vi "Dispatch Worker Mode Example(Sync).vi"() -> ()   [LabVIEW 2014]
uses:
  user.lib/_NEVSTOP/JKI State Machine ++/_Support/JKISMQ/_JKISMQFGV.vi
  user.lib/_NEVSTOP/JKI State Machine ++/JKI-State-Machine-Plus.lvlib
panel:
  in  "DoSth: DoA -@ Worker":bool
  in  "Name(\"\" to use uuid)":string="Event JKISM"
  out "State History":string
  in  "DoSth: DoA -> Worker":bool
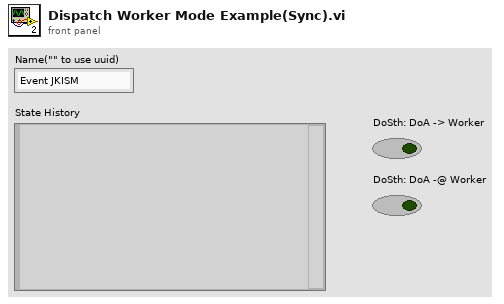
[diagram p1: front panel]
types:
  T1 = enum32{"Invalid", "Standard", "Closed", "Hidden", "Minimized", "Maximized"}
  T2 = enum32{"invalid app kind", "Development System", "Run Time System", "Student Edition", "Embedded LabVIEW", "Evaluation", "Custom"}
  T3 = cluster{"Core":cluster{"Current VI Reference":refnum<vi>, "Close Panel on Exit?":bool}, "Your Boolean data":bool, "Your string data":string}
  T4 = cluster{"Current VI Reference":refnum<vi>, "Close Panel on Exit?":bool}
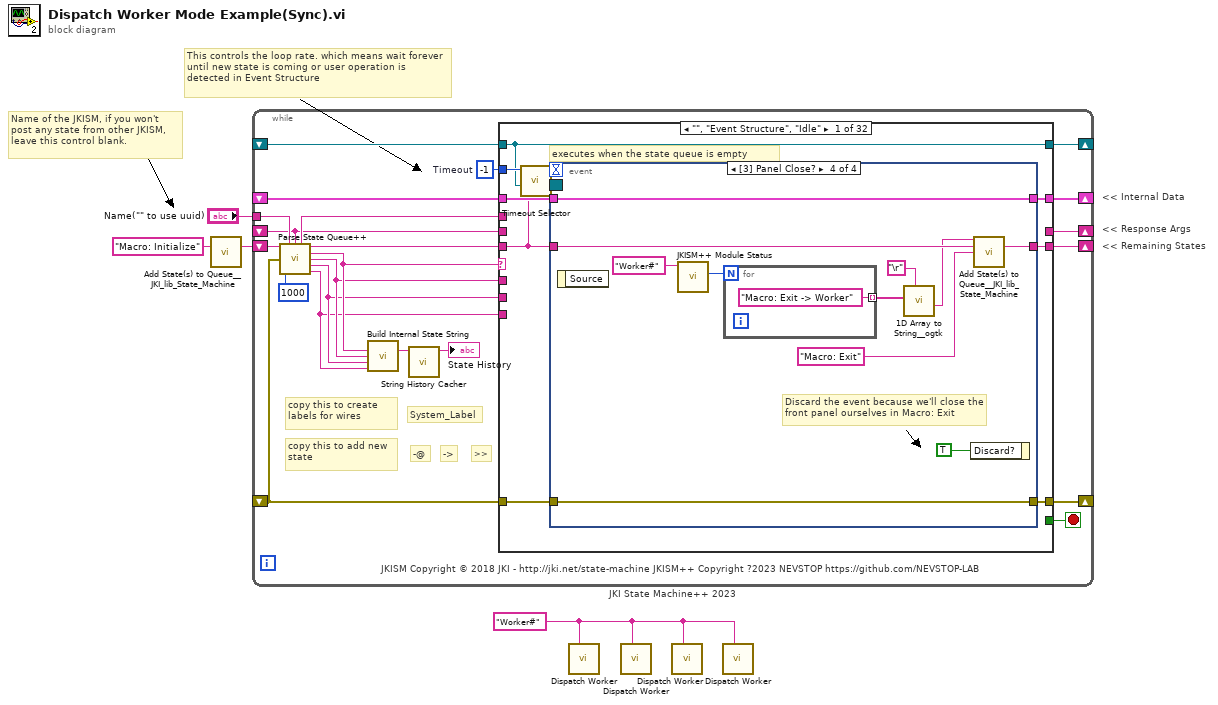
[diagram p0: block diagram]
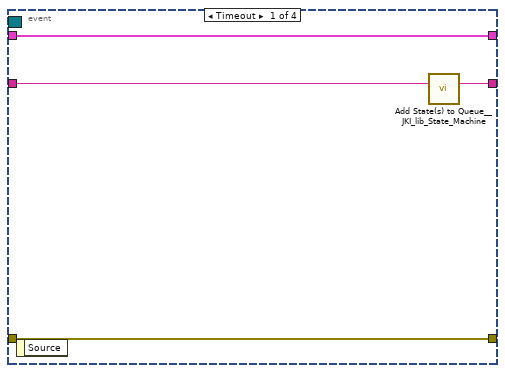
[diagram p2: hidden frame]
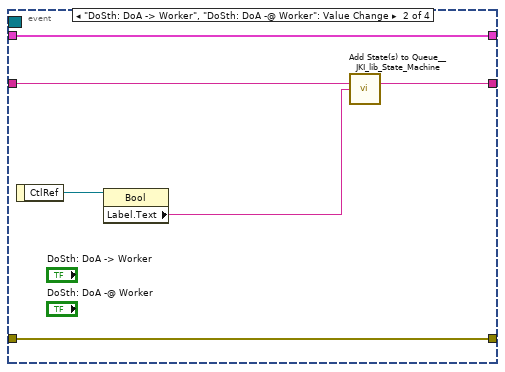
[diagram p3: hidden frame]
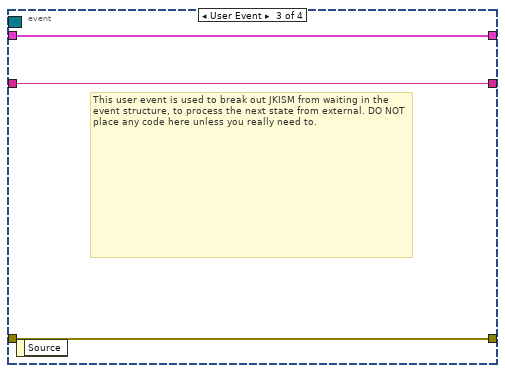
[diagram p4: hidden frame]
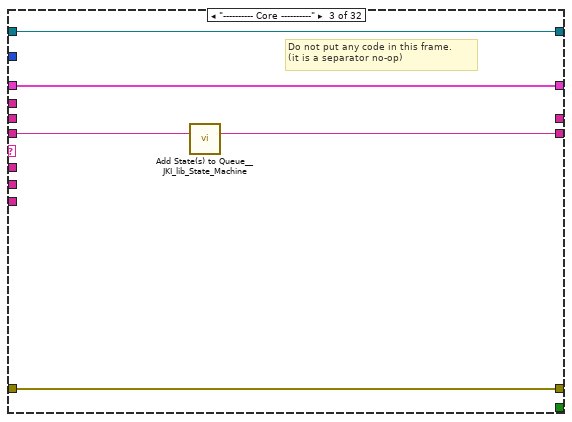
[diagram p6: hidden frame]
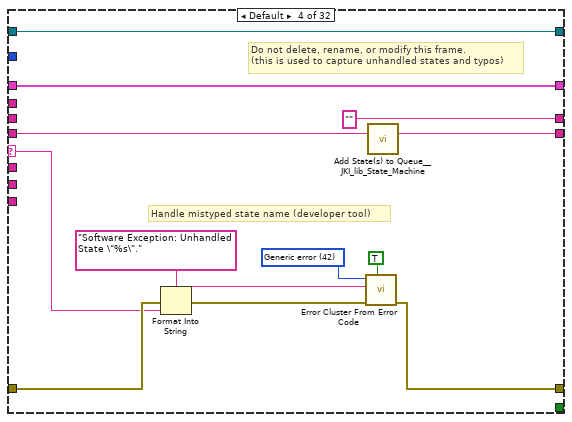
[diagram p7: hidden frame]
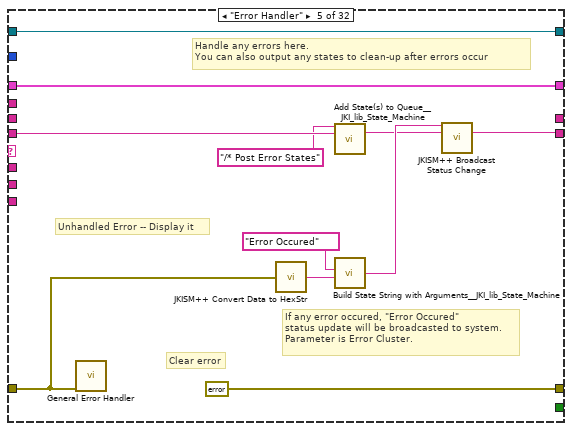
[diagram p8: hidden frame]
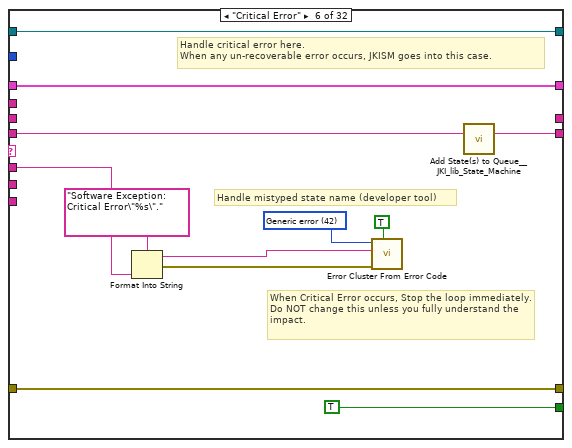
[diagram p9: hidden frame]
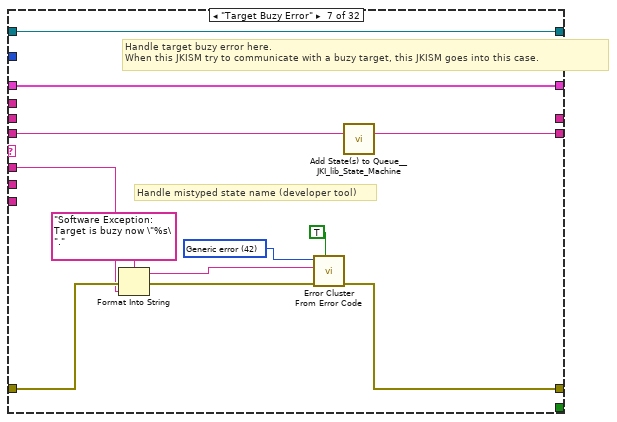
[diagram p10: hidden frame]
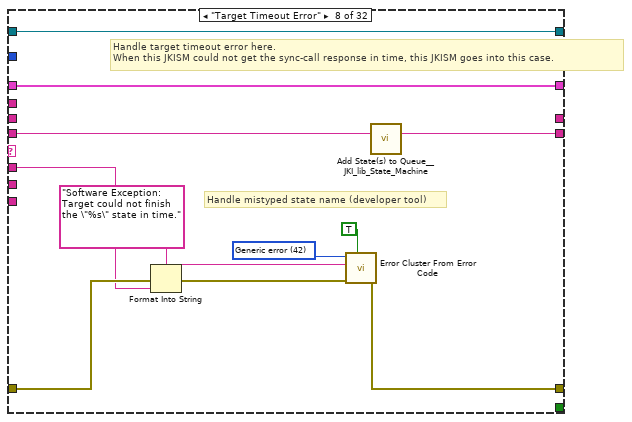
[diagram p11: hidden frame]
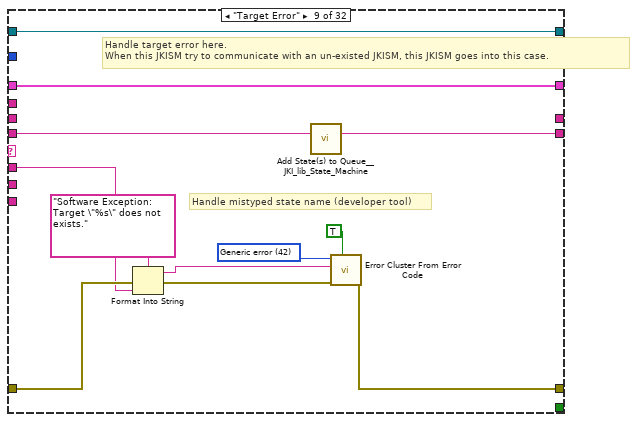
[diagram p12: hidden frame]
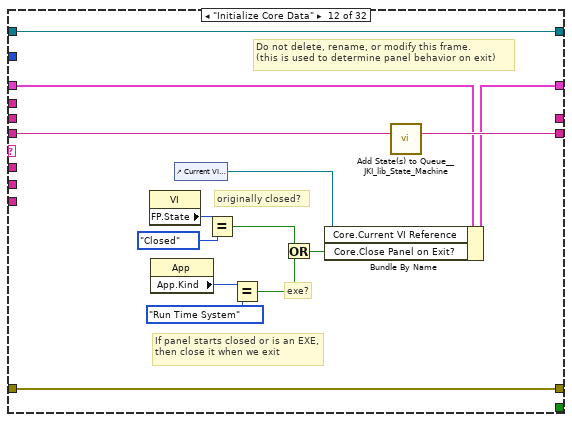
[diagram p15: hidden frame]
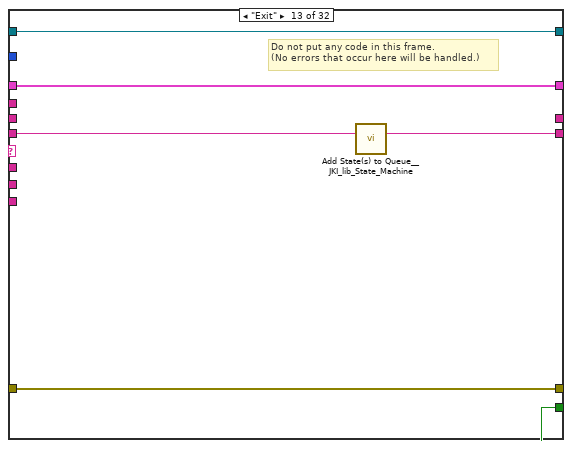
[diagram p16: hidden frame]
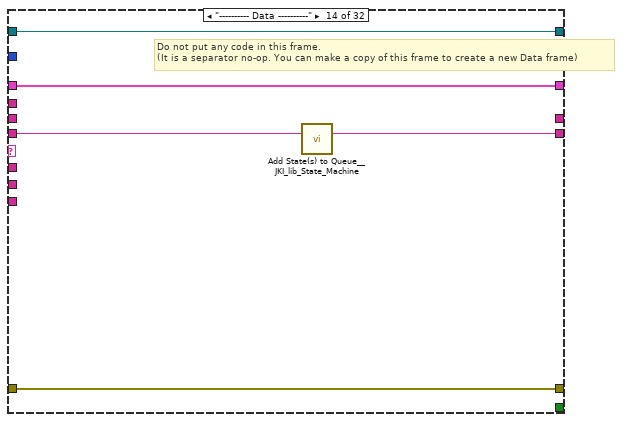
[diagram p17: hidden frame]
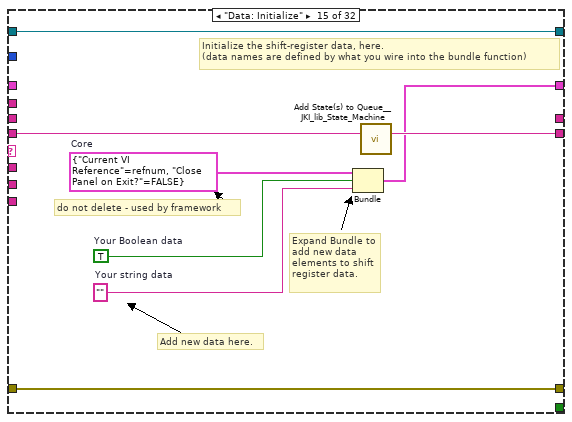
[diagram p18: hidden frame]
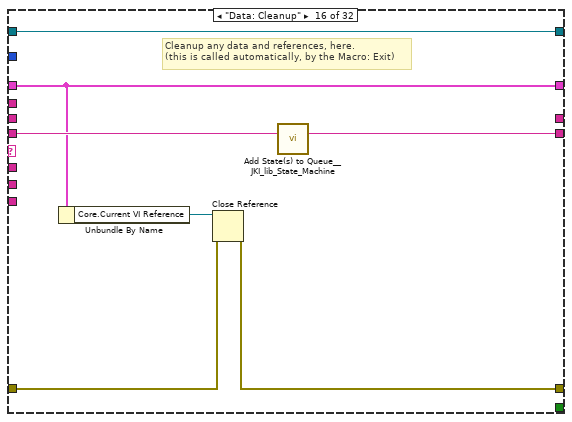
[diagram p19: hidden frame]
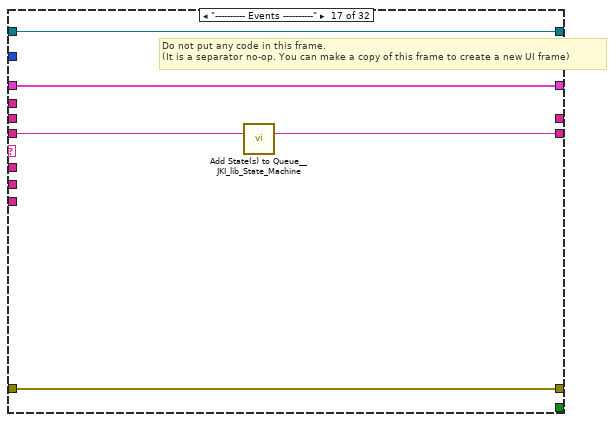
[diagram p20: hidden frame]
diagram:
  w1 = "Worker#" ("Name(\"\" to use uuid)")
  # "Name of the JKISM, if you won't post any state from other JKISM,  leave this control blank."
  # "This controls the loop rate. which means wait forever until new state is coming or user operation is detected in Event Structure"
  # "<< Internal Data"
  # "<< Response Args"
  # "<< Remaining States"
  n1 = call <vilib>:"Add State(s) to Queue__JKI_lib_State_Machine.vi"("State(s) in (\"\")"="Macro: Initialize") -> ("States Out"=w4:string)  [unwired: 14 in]
  n2 = while "JKI State Machine++ 2023" {
    shift-right: [w21] -> _
    shift-left: _ -> [w20]
    shift-right: [w24] -> _
    shift-left: _ -> [w18]
    shift-right: [w23] -> _
    shift-left: w4 -> [w25]
    tunnel: "Name(\"\" to use uuid)" -> [w13]
    shift-right: [w16] -> _
    shift-left: _ -> [w5]
    shift-right: [w15] -> _
    shift-left: _ -> [w14]
    stop <- w22 stop-if-true
    w19 = -1  # Timeout
    # "JKISM Copyright © 2018 JKI - http://jki.net/state-machine JKISM++ Copyright ?2023 NEVSTOP https://github.com/NEVSTOP-LAB"
    # "copy this to add new state"
    # ">>"
    # "->"
    # "-@"
    # "copy this to create labels for wires"
    # "System_Label"
    n3 = call "Parse State Queue++.vi"("State Queue"=w25, "Name(\"\" to use uuid)"=w13, "Response Arguments"=w5, "Error In (no error)"=w18, "Response Timeout(5000ms)"=1000 ("Response Timeout(1000ms)")) -> ("Name Used"=w6:string, "Remaining States"=w26:string, "Current State"=w10:string, "Arguments"=w9:string, "Argument - State"=w8:string, "From Who"=w7:string)  [unwired: 5 in]
    n4 = call "Build Internal State String.vi"("State"=w10, "Arguments (\"\")"=w9, "Arg-State (\"\")"=w8, "Source (\"\")"=w7) -> ("State with Arguments"=w11:string)  [unwired: 11 in]
    n5 = call "String History Cacher.vi"("String"=w11) -> ("String Cache"=→"State History":string)  [unwired: 10 in]
    n6 = case shown="\"\", \"Event Structure\", \"Idle\"" w10 {
      selector: w10 -> [_ _ _ w72 _ _ _ _ _ _ _ _ _ _ _ _ _ _ _ _ _ _ _ _ _ _ _ _ _ _ _ _]
      tunnel: w26 -> [w27 w63 w69 w76 w93 w103 w106 w123 w135 w144 w148 w163 w169 w174 w182 w189 w194 w200 w204 w210 w215 w222 w238 w308 w314 w325 w328 w333 w339 w347 w353 w359]
      tunnel: w9 -> [_ _ _ _ _ w96 w108 w119 w131 _ _ _ _ _ _ _ _ _ _ _ _ w217 w232 _ _ _ _ _ w336 _ _ _]
      tunnel: w20 -> [w34 w62 w66 w74 w91 w104 w110 w121 w133 w143 w147 w156 w167 w171 _ w184 w191 w199 w203 w207 w213 w220 w234 w305 w311 w322 w327 w332 w338 w344 w350 w356]
      tunnel: [w33 w64 w67 w78 errorcluster {"status"=FALSE, "code"=0, "source"=""} ("error out") w105 w113 w125 w137 w145 w149 w160 w166 w172 w179 w185 w192 w195 w202 w208 w212 w218 w235 w306 w312 w323 w329 w334 w340 w345 w351 w357] -> w24
      tunnel: w18 -> [w32 w64 w67 w77 w83 w105 w112 w124 w136 w145 w149 w160 w166 w172 w179 w186 w192 _ w205 w208 w212 w219 w236 w306 w312 w323 w329 w334 w340 w345 w351 w357]
      tunnel: [w35 w63 w68 w75 w84 w102 w111 w122 w134 w144 w148 w162 w168 w173 w181 w188 w193 w200 w204 w209 w214 w221 w237 w307 w313 w324 w328 w333 w339 w346 w352 w358] -> w23
      tunnel: [_ _ _ _ _ TRUE _ _ _ _ _ _ TRUE _ _ _ _ _ _ _ _ _ _ _ _ _ _ _ _ _ _ _] -> w22
      tunnel: [w31 w62 w66 w74 w91 w104 w110 w121 w133 w143 w147 w161 w167 w171 w180 w184 w191 w199 w203 w207 w213 w220 w234 w305 w311 w322 w327 w332 w338 w344 w350 w356] -> w21
      tunnel: w19 -> [w30 _ _ _ _ _ _ _ _ _ _ _ _ _ _ _ _ _ _ _ _ _ _ _ _ _ _ _ _ _ _ _]
      tunnel: w7 -> [_ _ _ _ _ _ _ _ _ _ _ _ _ _ _ _ _ _ _ _ _ _ _ _ _ _ _ _ _ _ _ _]
      tunnel: w8 -> [_ _ _ _ _ _ _ _ _ _ _ _ _ _ _ _ _ _ _ _ _ _ _ _ _ _ _ _ _ _ _ _]
      tunnel: [_ _ _ "" _ _ _ _ _ _ _ _ _ _ _ _ _ _ _ _ _ _ _ _ _ _ _ "API1 Response" w335 _ "DoA Finished" "DoB Finished"] -> w16
      tunnel: [w29 w61 w65 w70 w89 w94 w107 w118 w130 w142 w146 w150 w164 w170 w175 w183 w190 w198 w201 w206 w211 w216 w231 w304 w309 w315 w326 w331 w337 w343 w349 w355] -> w15
      tunnel: w14 -> [w29 w61 w65 w70 w89 w94 w107 w118 w130 w142 w146 w150 w164 w170 w175 w183 w190 _ w201 w206 w211 w216 w231 w304 w309 w315 w326 w331 w337 w343 w349 w355]
      tunnel: w6 -> [_ _ _ _ _ _ _ _ _ _ _ _ _ _ _ _ _ w197 _ _ _ _ _ _ _ _ _ _ _ _ _ _]
      tunnel: w5 -> [_ _ _ _ _ _ _ _ _ _ _ _ _ _ _ _ _ _ _ _ _ _ _ _ _ _ _ _ _ _ _ _]
      frame "", "Event Structure", "Idle" {
        # "executes when the state queue is empty"
        n7 = call "Timeout Selector.vi"("Remaining States"=w27, "Timeout Expected"=w30) -> ("Timeout"=w28:i32)  [unwired: 5 in]
        n8 = event shown="[3] Panel Close?" {
          selector: w29 -> [_ _ _ _]
          dyn-events: _ -> [_ _ _ _]
          timeout: w28 -> [_ _ _ _]
          tunnel: w27 -> [w39 w43 w47 w59]
          tunnel: [w38 w42 w47 w58] -> w35
          tunnel: w34 -> [w36 w44 w48 w56]
          tunnel: [w37 w45 w46 w57] -> w33
          tunnel: w32 -> [w37 w45 w46 w57]
          tunnel: [w36 w44 w48 w56] -> w31
          event Timeout {
            n9 = event-data() -> ()  [unwired: 1 in, 1 out]
            n10 = call <vilib>:"Add State(s) to Queue__JKI_lib_State_Machine.vi"("State(s) in (\"\")"=w39) -> ("States Out"=w38:string)  [unwired: 14 in]
          }
          event "DoSth: DoA -> Worker", "DoSth: DoA -@ Worker": Value Change {
            n11 = event-data() -> ("CtlRef"=w41:refnum<vi>)  [unwired: 1 in]
            n12 = property class="Bool"(reference=w41) -> ("Label.Text"=w40:string)  [unwired: 1 in, 2 out]
            n13 = call <vilib>:"Add State(s) to Queue__JKI_lib_State_Machine.vi"("State(s) in (\"\")"=w43, "State(s) at Back (\"\")"=w40) -> ("States Out"=w42:string)  [unwired: 13 in]
          }
          event User Event {
            # "This user event is used to break out JKISM from waiting in the event structure, to process the next state from external. DO NOT place any code here unless you really need to."
            n14 = event-data() -> ()  [unwired: 1 in, 1 out]
          }
          event Panel Close? {
            # "Discard the event because we'll close the front panel ourselves in Macro: Exit"
            n15 = event-data() -> ()  [unwired: 1 in, 1 out]
            n16 = call "JKISM++ Module Status.vi"("Name(\"\" to use uuid) in"="Worker#" ("Name(\"\" to use uuid)")) -> ("#AsWorker"=w53:i32)  [unwired: 7 in, 3 out]
            n17 = for {
              N: w53 -> [_]
              tunnel: ["Macro: Exit -> Worker"] -> w52 mode=indexing
            }
            n18 = call <userlib>:"1D Array to String__ogtk.vi"("delimiter (Tab)"="\r", "Array of Strings"=w52) -> ("delimited string"=w51:string)  [unwired: 9 in]
            n19 = event-data("Discard?"=TRUE) -> ()  [unwired: 1 in, 1 out]
            n20 = call <vilib>:"Add State(s) to Queue__JKI_lib_State_Machine.vi"("State(s) in Front (\"\")"=w51, "State(s) in (\"\")"=w59, "State(s) at Back (\"\")"="Macro: Exit") -> ("States Out"=w58:string)  [unwired: 12 in]
          }
        }
      }
      frame "JKISM++ Documentation" {
        # "JKISM++ Documentation"
        # "State Syntax:\nStateCategory: State >> Argument -@ JKISMName\nStateCategory: State >> Argument -> JKISMName\n\nLine Terminator: Line feed"
        # "Commenting:\nTo add a comment use \"//\" or \"#\" and all text to the right will be ignored\nCommenting Example:\nUI: Initialize // This initializes the UI\n# This whole line is a comment\n// Another comment line"
      }
      frame "---------- Core ----------" {
        # "Do not put any code in this frame.\n(it is a separator no-op)"
        n21 = call <vilib>:"Add State(s) to Queue__JKI_lib_State_Machine.vi"("State(s) in (\"\")"=w69) -> ("States Out"=w68:string)  [unwired: 14 in]
      }
      frame Default {
        w81 = 42 items=["No error", "Argument error", "Memory is full", "Out of zone", "End of file", "File already open", "Generic file I/O error", "File not found", "File permission error", "Disk is full", "Duplicate path", "Too many files open", "System feature not enabled", "Resource file not found", "Cannot add resource", "Resource not found", "Image not found", "Image memory error", "Pen does not exist", "Config type invalid", "Config token not found", "Config parse error", "Config memory error", "Bad external code format", "Bad external code offset", "External code not present", "Null window", "Destroy window error", "Null menu", "Print aborted", "Bad print record", "Print driver error", "Windows error during printing", "Memory error during printing", "Print dialog error", "Generic print error", "Invalid device refnum", "Device not found", "Device parameter error", "Device unit error", "Cannot open device", "Device call aborted", "Generic error", "Cancelled by user", "Object ID too low", "Object ID too high", "Object not in heap", "Unknown heap", "Unknown object (invalid DefProc)", "Unknown object (DefProc not in table)", "Message out of range", "Invalid (null) method", "Unknown message", "Manager call not supported", "Bad address", "Network operation in progress", "Network operation timed out", "Connection is busy", "Network attribute not supported", "Network error", "Address in use", "System out of memory", "Connection aborted", "Connection refused", "Not connected", "Already connected", "Connection closed", "Initialization error (interapplication manager)", "Bad occurrence", "Wait on unbound occurrence handler", "Occurrence queue overflow", "Datalog type conflict", "Unused", "Unrecognized type (interapplication manager)", "Memory corrupt", "Failed to make temporary DLL", "Old CIN version", "Drag socket not found", "Failed to load drop-object", "Failed to register OLE object", "Failed to release OLE object", "Format specifier type mismatch", "Unknown format specifier", "Too few format specifiers", "Too many format specifiers", "Scan failed", "Newer CIN version", "Error converting to variant", "Runtime menu error", "Password tampered", "Variant attribute not found", "Incompatible variant data type", "Event data is not available", "Event Store is not present", "Occurrence is not found", "Event Queue is not created", "Event info is not available", "Refnum passed is NULL", "Error retrieving Class GUID", "Error retrieving CoClass GUID", "Error retrieving TypeLib GUID.", "Bad built application magic bytes.", "Specific driver is different from the specific driver associated with the Logical Name.", "There is no session opened to the class driver.", "Max Error", "MAX - Error with config objects", "MAX - Error loading configuration", "MAX - Group not supported"]
        # "Do not delete, rename, or modify this frame.\n(this is used to capture unhandled states and typos)"
        # "Handle mistyped state name (developer tool)"
        n22 = Format Into String(format string="Software Exception: Unhandled State \"%s\"." ("message"), error in=w77, w72) -> (resulting string=w80:string, error out=w79:errorcluster)  [unwired: 1 in]
        n23 = call <vilib>:"Error Cluster From Error Code.vi"("show call chain? (False)"=TRUE, "error in (no error)"=w79, "error message (\"\")"=w80, "error code (0)"=w81) -> ("error out"=w78:errorcluster)  [unwired: 5 in]
        n24 = call <vilib>:"Add State(s) to Queue__JKI_lib_State_Machine.vi"("State(s) in (\"\")"=w76) -> ("States Out"=w75:string)  [unwired: 14 in]
      }
      frame "Error Handler" {
        # "If any error occured, \"Error Occured\" \nstatus update will be broadcasted to system.\nParameter is Error Cluster."
        # "Unhandled Error -- Display it"
        # "Handle any errors here.\nYou can also output any states to clean-up after errors occur"
        # "Clear error"
        n25 = call <vilib>:"General Error Handler.vi"("error in (no error)"=w83) -> ()  [unwired: 10 in, 5 out]
        n26 = call "JKISM++ Convert Data to HexStr.vi"("Variant"=w83) -> ("HEX String (0-9,A-F)"=w87:string)  [unwired: 8 in]
        n27 = call <vilib>:"Add State(s) to Queue__JKI_lib_State_Machine.vi"("State(s) in Front (\"\")"="/* Post Error States", "State(s) in (\"\")"=w93) -> ("States Out"=w85:string)  [unwired: 13 in]
        n28 = call <vilib>:"Build State String with Arguments__JKI_lib_State_Machine.vi"("Arguments (\"\")"=w87, "State"="Error Occured" ("Status with Arguments")) -> ("State with Arguments"=w86:string)  [unwired: 4 in]
        n29 = call "JKISM++ Broadcast Status Change.vi"("Status with Arguments"=w86, "State(s) in (\"\")"=w85) -> ("States Out"=w84:string)  [unwired: 13 in]
      }
      frame "Critical Error" {
        w100 = 42 items=["No error", "Argument error", "Memory is full", "Out of zone", "End of file", "File already open", "Generic file I/O error", "File not found", "File permission error", "Disk is full", "Duplicate path", "Too many files open", "System feature not enabled", "Resource file not found", "Cannot add resource", "Resource not found", "Image not found", "Image memory error", "Pen does not exist", "Config type invalid", "Config token not found", "Config parse error", "Config memory error", "Bad external code format", "Bad external code offset", "External code not present", "Null window", "Destroy window error", "Null menu", "Print aborted", "Bad print record", "Print driver error", "Windows error during printing", "Memory error during printing", "Print dialog error", "Generic print error", "Invalid device refnum", "Device not found", "Device parameter error", "Device unit error", "Cannot open device", "Device call aborted", "Generic error", "Cancelled by user", "Object ID too low", "Object ID too high", "Object not in heap", "Unknown heap", "Unknown object (invalid DefProc)", "Unknown object (DefProc not in table)", "Message out of range", "Invalid (null) method", "Unknown message", "Manager call not supported", "Bad address", "Network operation in progress", "Network operation timed out", "Connection is busy", "Network attribute not supported", "Network error", "Address in use", "System out of memory", "Connection aborted", "Connection refused", "Not connected", "Already connected", "Connection closed", "Initialization error (interapplication manager)", "Bad occurrence", "Wait on unbound occurrence handler", "Occurrence queue overflow", "Datalog type conflict", "Unused", "Unrecognized type (interapplication manager)", "Memory corrupt", "Failed to make temporary DLL", "Old CIN version", "Drag socket not found", "Failed to load drop-object", "Failed to register OLE object", "Failed to release OLE object", "Format specifier type mismatch", "Unknown format specifier", "Too few format specifiers", "Too many format specifiers", "Scan failed", "Newer CIN version", "Error converting to variant", "Runtime menu error", "Password tampered", "Variant attribute not found", "Incompatible variant data type", "Event data is not available", "Event Store is not present", "Occurrence is not found", "Event Queue is not created", "Event info is not available", "Refnum passed is NULL", "Error retrieving Class GUID", "Error retrieving CoClass GUID", "Error retrieving TypeLib GUID.", "Bad built application magic bytes.", "Specific driver is different from the specific driver associated with the Logical Name.", "There is no session opened to the class driver.", "Max Error", "MAX - Error with config objects", "MAX - Error loading configuration", "MAX - Group not supported"]
        # "Handle critical error here.\nWhen any un-recoverable error occurs, JKISM goes into this case."
        # "When Critical Error occurs, Stop the loop immediately. Do NOT change this unless you fully understand the impact."
        # "Handle mistyped state name (developer tool)"
        n30 = Format Into String(format string="Software Exception: Critical Error\"%s\"." ("message"), w96) -> (resulting string=w99:string, error out=w98:errorcluster)  [unwired: 2 in]
        n31 = call <vilib>:"Error Cluster From Error Code.vi"("show call chain? (False)"=TRUE, "error in (no error)"=w98, "error message (\"\")"=w99, "error code (0)"=w100) -> ()  [unwired: 5 in, 1 out]
        n32 = call <vilib>:"Add State(s) to Queue__JKI_lib_State_Machine.vi"("State(s) in (\"\")"=w103) -> ("States Out"=w102:string)  [unwired: 14 in]
      }
      frame "Target Buzy Error" {
        w116 = 42 items=["No error", "Argument error", "Memory is full", "Out of zone", "End of file", "File already open", "Generic file I/O error", "File not found", "File permission error", "Disk is full", "Duplicate path", "Too many files open", "System feature not enabled", "Resource file not found", "Cannot add resource", "Resource not found", "Image not found", "Image memory error", "Pen does not exist", "Config type invalid", "Config token not found", "Config parse error", "Config memory error", "Bad external code format", "Bad external code offset", "External code not present", "Null window", "Destroy window error", "Null menu", "Print aborted", "Bad print record", "Print driver error", "Windows error during printing", "Memory error during printing", "Print dialog error", "Generic print error", "Invalid device refnum", "Device not found", "Device parameter error", "Device unit error", "Cannot open device", "Device call aborted", "Generic error", "Cancelled by user", "Object ID too low", "Object ID too high", "Object not in heap", "Unknown heap", "Unknown object (invalid DefProc)", "Unknown object (DefProc not in table)", "Message out of range", "Invalid (null) method", "Unknown message", "Manager call not supported", "Bad address", "Network operation in progress", "Network operation timed out", "Connection is busy", "Network attribute not supported", "Network error", "Address in use", "System out of memory", "Connection aborted", "Connection refused", "Not connected", "Already connected", "Connection closed", "Initialization error (interapplication manager)", "Bad occurrence", "Wait on unbound occurrence handler", "Occurrence queue overflow", "Datalog type conflict", "Unused", "Unrecognized type (interapplication manager)", "Memory corrupt", "Failed to make temporary DLL", "Old CIN version", "Drag socket not found", "Failed to load drop-object", "Failed to register OLE object", "Failed to release OLE object", "Format specifier type mismatch", "Unknown format specifier", "Too few format specifiers", "Too many format specifiers", "Scan failed", "Newer CIN version", "Error converting to variant", "Runtime menu error", "Password tampered", "Variant attribute not found", "Incompatible variant data type", "Event data is not available", "Event Store is not present", "Occurrence is not found", "Event Queue is not created", "Event info is not available", "Refnum passed is NULL", "Error retrieving Class GUID", "Error retrieving CoClass GUID", "Error retrieving TypeLib GUID.", "Bad built application magic bytes.", "Specific driver is different from the specific driver associated with the Logical Name.", "There is no session opened to the class driver.", "Max Error", "MAX - Error with config objects", "MAX - Error loading configuration", "MAX - Group not supported"]
        # "Handle target buzy error here.\nWhen this JKISM try to communicate with a buzy target, this JKISM goes into this case."
        # "Handle mistyped state name (developer tool)"
        n33 = Format Into String(format string="Software Exception: Target is buzy now \"%s\"." ("message"), error in=w112, w108) -> (resulting string=w115:string, error out=w114:errorcluster)  [unwired: 1 in]
        n34 = call <vilib>:"Error Cluster From Error Code.vi"("show call chain? (False)"=TRUE, "error in (no error)"=w114, "error message (\"\")"=w115, "error code (0)"=w116) -> ("error out"=w113:errorcluster)  [unwired: 5 in]
        n35 = call <vilib>:"Add State(s) to Queue__JKI_lib_State_Machine.vi"("State(s) in (\"\")"=w106) -> ("States Out"=w111:string)  [unwired: 14 in]
      }
      frame "Target Timeout Error" {
        w128 = 42 items=["No error", "Argument error", "Memory is full", "Out of zone", "End of file", "File already open", "Generic file I/O error", "File not found", "File permission error", "Disk is full", "Duplicate path", "Too many files open", "System feature not enabled", "Resource file not found", "Cannot add resource", "Resource not found", "Image not found", "Image memory error", "Pen does not exist", "Config type invalid", "Config token not found", "Config parse error", "Config memory error", "Bad external code format", "Bad external code offset", "External code not present", "Null window", "Destroy window error", "Null menu", "Print aborted", "Bad print record", "Print driver error", "Windows error during printing", "Memory error during printing", "Print dialog error", "Generic print error", "Invalid device refnum", "Device not found", "Device parameter error", "Device unit error", "Cannot open device", "Device call aborted", "Generic error", "Cancelled by user", "Object ID too low", "Object ID too high", "Object not in heap", "Unknown heap", "Unknown object (invalid DefProc)", "Unknown object (DefProc not in table)", "Message out of range", "Invalid (null) method", "Unknown message", "Manager call not supported", "Bad address", "Network operation in progress", "Network operation timed out", "Connection is busy", "Network attribute not supported", "Network error", "Address in use", "System out of memory", "Connection aborted", "Connection refused", "Not connected", "Already connected", "Connection closed", "Initialization error (interapplication manager)", "Bad occurrence", "Wait on unbound occurrence handler", "Occurrence queue overflow", "Datalog type conflict", "Unused", "Unrecognized type (interapplication manager)", "Memory corrupt", "Failed to make temporary DLL", "Old CIN version", "Drag socket not found", "Failed to load drop-object", "Failed to register OLE object", "Failed to release OLE object", "Format specifier type mismatch", "Unknown format specifier", "Too few format specifiers", "Too many format specifiers", "Scan failed", "Newer CIN version", "Error converting to variant", "Runtime menu error", "Password tampered", "Variant attribute not found", "Incompatible variant data type", "Event data is not available", "Event Store is not present", "Occurrence is not found", "Event Queue is not created", "Event info is not available", "Refnum passed is NULL", "Error retrieving Class GUID", "Error retrieving CoClass GUID", "Error retrieving TypeLib GUID.", "Bad built application magic bytes.", "Specific driver is different from the specific driver associated with the Logical Name.", "There is no session opened to the class driver.", "Max Error", "MAX - Error with config objects", "MAX - Error loading configuration", "MAX - Group not supported"]
        # "Handle target timeout error here.\nWhen this JKISM could not get the sync-call response in time, this JKISM goes into this case."
        # "Handle mistyped state name (developer tool)"
        n36 = Format Into String(format string="Software Exception: Target could not finish the \"%s\" state in time." ("message"), error in=w124, w119) -> (resulting string=w127:string, error out=w126:errorcluster)  [unwired: 1 in]
        n37 = call <vilib>:"Error Cluster From Error Code.vi"("show call chain? (False)"=TRUE, "error in (no error)"=w126, "error message (\"\")"=w127, "error code (0)"=w128) -> ("error out"=w125:errorcluster)  [unwired: 5 in]
        n38 = call <vilib>:"Add State(s) to Queue__JKI_lib_State_Machine.vi"("State(s) in (\"\")"=w123) -> ("States Out"=w122:string)  [unwired: 14 in]
      }
      frame "Target Error" {
        w140 = 42 items=["No error", "Argument error", "Memory is full", "Out of zone", "End of file", "File already open", "Generic file I/O error", "File not found", "File permission error", "Disk is full", "Duplicate path", "Too many files open", "System feature not enabled", "Resource file not found", "Cannot add resource", "Resource not found", "Image not found", "Image memory error", "Pen does not exist", "Config type invalid", "Config token not found", "Config parse error", "Config memory error", "Bad external code format", "Bad external code offset", "External code not present", "Null window", "Destroy window error", "Null menu", "Print aborted", "Bad print record", "Print driver error", "Windows error during printing", "Memory error during printing", "Print dialog error", "Generic print error", "Invalid device refnum", "Device not found", "Device parameter error", "Device unit error", "Cannot open device", "Device call aborted", "Generic error", "Cancelled by user", "Object ID too low", "Object ID too high", "Object not in heap", "Unknown heap", "Unknown object (invalid DefProc)", "Unknown object (DefProc not in table)", "Message out of range", "Invalid (null) method", "Unknown message", "Manager call not supported", "Bad address", "Network operation in progress", "Network operation timed out", "Connection is busy", "Network attribute not supported", "Network error", "Address in use", "System out of memory", "Connection aborted", "Connection refused", "Not connected", "Already connected", "Connection closed", "Initialization error (interapplication manager)", "Bad occurrence", "Wait on unbound occurrence handler", "Occurrence queue overflow", "Datalog type conflict", "Unused", "Unrecognized type (interapplication manager)", "Memory corrupt", "Failed to make temporary DLL", "Old CIN version", "Drag socket not found", "Failed to load drop-object", "Failed to register OLE object", "Failed to release OLE object", "Format specifier type mismatch", "Unknown format specifier", "Too few format specifiers", "Too many format specifiers", "Scan failed", "Newer CIN version", "Error converting to variant", "Runtime menu error", "Password tampered", "Variant attribute not found", "Incompatible variant data type", "Event data is not available", "Event Store is not present", "Occurrence is not found", "Event Queue is not created", "Event info is not available", "Refnum passed is NULL", "Error retrieving Class GUID", "Error retrieving CoClass GUID", "Error retrieving TypeLib GUID.", "Bad built application magic bytes.", "Specific driver is different from the specific driver associated with the Logical Name.", "There is no session opened to the class driver.", "Max Error", "MAX - Error with config objects", "MAX - Error loading configuration", "MAX - Group not supported"]
        # "Handle target error here.\nWhen this JKISM try to communicate with an un-existed JKISM, this JKISM goes into this case."
        # "Handle mistyped state name (developer tool)"
        n39 = Format Into String(format string="Software Exception: Target \"%s\" does not exists." ("message"), error in=w136, w131) -> (resulting string=w139:string, error out=w138:errorcluster)  [unwired: 1 in]
        n40 = call <vilib>:"Add State(s) to Queue__JKI_lib_State_Machine.vi"("State(s) in (\"\")"=w135) -> ("States Out"=w134:string)  [unwired: 14 in]
        n41 = call <vilib>:"Error Cluster From Error Code.vi"("show call chain? (False)"=TRUE, "error in (no error)"=w138, "error message (\"\")"=w139, "error code (0)"=w140) -> ("error out"=w137:errorcluster)  [unwired: 5 in]
      }
      frame "Async Response", "Response" {
        # "Handle Async-call Response (\"Async Response\" for ->)"
        # "Handle Sync-call Response (\"Response\" for @)"
        # "After Message is excuted, JKISM+ goes to this state for recieve the response. \n    For Async Message(->), \"Async Response\" is used. This JKISM will goes to \"Async Message Posted\" immediately and recieve the \"Async Response\" after the callee finishes the message.\n    For Sync Message(@),  This JKISM will wait until the message is done and immidieatly goes to \"Response\""
      }
      frame "Async Message Posted" {
        # "Handle post action for async message (->)."
        # "After Async Message is posted (->), JKISM+ goes to this state for post-action. You can use Argument - State to tell which Async Message is called."
      }
      frame "Initialize Core Data" {
        # "Do not delete, rename, or modify this frame.\n(this is used to determine panel behavior on exit)"
        # "originally closed?"
        # "exe?"
        # "If panel starts closed or is an EXE, then close it when we exit"
        n42 = property class="VI"() -> ("FP.State"=w153:T1)  [unwired: 2 in, 2 out]
        n43 = property class="App"() -> ("App.Kind"=w159:T2)  [unwired: 2 in, 2 out]
        n44 = control-ref of="Current VI Reference"() -> (w154:refnum<vi>)
        n45 = Equal?(x=w153, y=T1."Closed" ("Front Panel Window:State")) -> (x = y?=w151:bool)
        n46 = Equal?(x=w159, y=T2."Run Time System" ("Application:Kind")) -> (x = y?=w157:bool)
        n47 = Or(x=w151, y=w157) -> (x .or. y?=w155:bool)
        n48 = Bundle By Name(cluster=w156, "Core.Current VI Reference"=w154, "Core.Close Panel on Exit?"=w155) -> (w161:T3)
        n49 = call <vilib>:"Add State(s) to Queue__JKI_lib_State_Machine.vi"("State(s) in (\"\")"=w163) -> ("States Out"=w162:string)  [unwired: 14 in]
      }
      frame "Exit" {
        # "Do not put any code in this frame.\n(No errors that occur here will be handled.)"
        n50 = call <vilib>:"Add State(s) to Queue__JKI_lib_State_Machine.vi"("State(s) in (\"\")"=w169) -> ("States Out"=w168:string)  [unwired: 14 in]
      }
      frame "---------- Data ----------" {
        # "Do not put any code in this frame.\n(It is a separator no-op. You can make a copy of this frame to create a new Data frame)"
        n51 = call <vilib>:"Add State(s) to Queue__JKI_lib_State_Machine.vi"("State(s) in (\"\")"=w174) -> ("States Out"=w173:string)  [unwired: 14 in]
      }
      frame "Data: Initialize" {
        w176 = T4 {"Current VI Reference"=refnum, "Close Panel on Exit?"=FALSE}  # Core
        w178 = TRUE  # Your Boolean data
        w177 = ""  # Your string data
        # "do not delete - used by framework"
        # "Expand Bundle to add new data elements to shift register data."
        # "Add new data here."
        # "Initialize the shift-register data, here.\n(data names are defined by what you wire into the bundle function)"
        n52 = Bundle("Core"=w176, "Your Boolean data"=w178, "Your string data"=w177) -> (w180:T3)  [unwired: 1 in]
        n53 = call <vilib>:"Add State(s) to Queue__JKI_lib_State_Machine.vi"("State(s) in (\"\")"=w182) -> ("States Out"=w181:string)  [unwired: 14 in]
      }
      frame "Data: Cleanup" {
        # "Cleanup any data and references, here.\n(this is called automatically, by the Macro: Exit)"
        n54 = Unbundle By Name(w184) -> ("Core.Current VI Reference"=w187:refnum<vi>)
        n55 = Close Reference(reference=w187, error in (no error)=w186) -> (error out=w185:errorcluster)
        n56 = call <vilib>:"Add State(s) to Queue__JKI_lib_State_Machine.vi"("State(s) in (\"\")"=w189) -> ("States Out"=w188:string)  [unwired: 14 in]
      }
      frame "---------- Events ----------" {
        # "Do not put any code in this frame.\n(It is a separator no-op. You can make a copy of this frame to create a new UI frame)"
        n57 = call <vilib>:"Add State(s) to Queue__JKI_lib_State_Machine.vi"("State(s) in (\"\")"=w194) -> ("States Out"=w193:string)  [unwired: 14 in]
      }
      frame "Events: Register" {
        # "Register message event to break Waiting in Event structure."
        n58 = call "JKISM++ Get New State Notifier Event.vi"("Name(\"\" to use uuid) in"=w197) -> ("Error out"=w195:errorcluster, "New State Notifier Event"=w196:refnum<user-event>)  [unwired: 9 in]
        n59 = register-events(w196) -> (reference out=w198:refnum<event-registration>)  [unwired: 2 in, 1 out]
      }
      frame "Events: Unregister" {
        n60 = Unregister For Events(event registration refnum=w201, error in=w205) -> (error out=w202:errorcluster)
      }
      frame "---------- UI ----------" {
        # "Do not put any code in this frame.\n(It is a separator no-op. You can make a copy of this frame to create a new UI frame)"
        n61 = call <vilib>:"Add State(s) to Queue__JKI_lib_State_Machine.vi"("State(s) in (\"\")"=w210) -> ("States Out"=w209:string)  [unwired: 14 in]
      }
      frame "UI: Initialize" {
        # "Initialize the User Interface, here.\n(this is called automatically, by the Macro: Init)"
        n62 = call <vilib>:"Add State(s) to Queue__JKI_lib_State_Machine.vi"("State(s) in (\"\")"=w215) -> ("States Out"=w214:string)  [unwired: 14 in]
      }
      frame "UI: Cursor Set" {
        # "Argument"
        # "Set and Unset Cursor Busy.\n(Usage: \"UI: Cursor Set >> Busy|Idle\")"
        n63 = disable-structure shown="TARGET_TYPE!=Windows" {
          disable-tunnel: w219 -> [w225 w230]
          disable-tunnel: [w224 w230] -> w218
          disable-tunnel: w217 -> [w223 _]
          frame condition #0 (active) {
            n64 = case shown="\"Idle\", Default" w223 {
              tunnel: w225 -> [w227 w229]
              tunnel: [w226 w228] -> w224
              frame "Idle", Default {
                n65 = call <vilib>:"Unset Busy.vi"("error in (no error)"=w227) -> ("error out"=w226:errorcluster)  [unwired: 10 in]
              }
              frame "Busy" {
                n66 = call <vilib>:"Set Busy.vi"("error in (no error)"=w229) -> ("error out"=w228:errorcluster)  [unwired: 9 in, 1 out]
              }
            }
          }
          frame condition #1 {
          }
        }
        n67 = call <vilib>:"Add State(s) to Queue__JKI_lib_State_Machine.vi"("State(s) in (\"\")"=w222) -> ("States Out"=w221:string)  [unwired: 14 in]
      }
      frame "UI: Front Panel State" {
        # "Argument"
        # "Set Front Panel Open or Closed\n(Usage: \"UI: Front Panel State >> Open|Close\")"
        n68 = Unbundle By Name(w234) -> ("Core.Current VI Reference"=w233:refnum<vi>)
        n69 = call <vilib>:"Add State(s) to Queue__JKI_lib_State_Machine.vi"("State(s) in (\"\")"=w238) -> ("States Out"=w237:string)  [unwired: 14 in]
        n70 = case shown="\"Minimize\", \"Minimized\"" w232 {
          tunnel: w236 -> [w244 w259 w270 w283 w296]
          tunnel: [w246 w260 w272 w285 w298] -> w235
          tunnel: w233 -> [w245 w257 w271 w284 w297]
          frame "Open", "Standard", Default {
            w239 = T1."Standard" ("State")
            n71 = property class="VI"(reference=w245, error in=w244) -> (reference out=w242:refnum<vi>, error out=w243:errorcluster, "FP.State"=w241:T1)
            n72 = Not Equal?(x=w241, y=w239) -> (x != y?=w240:bool)
            n73 = case shown="True" w240 {
              tunnel: [w250 w252] -> w246
              tunnel: w243 -> [w249 w252]
              tunnel: w242 -> [w248 _]
              tunnel: w239 -> [w247 _]
              frame True {
                n74 = invoke class="VI" method="FP.Open"(reference=w248, error in=w249, "Activate"=TRUE, "State"=w247) -> (error out=w250:errorcluster)  [unwired: 1 in, 4 out]
              }
              frame False {
              }
            }
          }
          frame "Close", "Closed" {
            n75 = property class="VI"(reference=w257, error in=w259) -> (reference out=w256:refnum<vi>, error out=w258:errorcluster, "FP.State"=w254:T1)
            n76 = Not Equal?(x=w254, y=T1."Closed" ("Front Panel Window:State")) -> (x != y?=w253:bool)
            n77 = case shown="True" w253 {
              tunnel: [w261 w264] -> w260
              tunnel: w258 -> [w261 w263]
              tunnel: w256 -> [_ w262]
              frame False {
              }
              frame True {
                n78 = invoke class="VI" method="FP.Close"(reference=w262, error in=w263) -> (error out=w264:errorcluster)  [unwired: 1 in, 2 out]
              }
            }
          }
          frame "Hidden", "Hide" {
            w265 = T1."Hidden" ("State")
            n79 = property class="VI"(reference=w271, error in=w270) -> (reference out=w268:refnum<vi>, error out=w269:errorcluster, "FP.State"=w267:T1)
            n80 = Not Equal?(x=w267, y=w265) -> (x != y?=w266:bool)
            n81 = case shown="True" w266 {
              tunnel: [w276 w277] -> w272
              tunnel: w269 -> [w275 w277]
              tunnel: w268 -> [w274 _]
              tunnel: w265 -> [w273 _]
              frame True {
                n82 = invoke class="VI" method="FP.Open"(reference=w274, error in=w275, "State"=w273) -> (error out=w276:errorcluster)  [unwired: 2 in, 4 out]
              }
              frame False {
              }
            }
          }
          frame "Minimize", "Minimized" {
            w278 = T1."Minimized" ("State")
            n83 = property class="VI"(reference=w284, error in=w283) -> (reference out=w281:refnum<vi>, error out=w282:errorcluster, "FP.State"=w280:T1)
            n84 = Not Equal?(x=w280, y=w278) -> (x != y?=w279:bool)
            n85 = case shown="True" w279 {
              tunnel: [w289 w290] -> w285
              tunnel: w282 -> [w288 w290]
              tunnel: w281 -> [w287 _]
              tunnel: w278 -> [w286 _]
              frame True {
                n86 = invoke class="VI" method="FP.Open"(reference=w287, error in=w288, "State"=w286) -> (error out=w289:errorcluster)  [unwired: 2 in, 4 out]
              }
              frame False {
              }
            }
          }
          frame "Maximize", "Maximized" {
            w291 = T1."Maximized" ("State")
            n87 = property class="VI"(reference=w297, error in=w296) -> (reference out=w294:refnum<vi>, error out=w295:errorcluster, "FP.State"=w293:T1)
            n88 = Not Equal?(x=w293, y=w291) -> (x != y?=w292:bool)
            n89 = case shown="True" w292 {
              tunnel: [w302 w303] -> w298
              tunnel: w295 -> [w301 w303]
              tunnel: w294 -> [w300 _]
              tunnel: w291 -> [w299 _]
              frame True {
                n90 = invoke class="VI" method="FP.Open"(reference=w300, error in=w301, "State"=w299) -> (error out=w302:errorcluster)  [unwired: 2 in, 4 out]
              }
              frame False {
              }
            }
          }
        }
      }
      frame "---------- Macro ----------" {
        # "Do not put any code in this frame.\n(It is a separator no-op. You can make a copy of this frame to create a new Macro frame)"
        n91 = call <vilib>:"Add State(s) to Queue__JKI_lib_State_Machine.vi"("State(s) in (\"\")"=w308) -> ("States Out"=w307:string)  [unwired: 14 in]
      }
      frame "Macro: Initialize" {
        w310 = "Data: Initialize\nInitialize Core Data\nEvents: Register\nUI: Initialize\nUI: Front Panel State >> Open"  # Data: Initialize Initialize Core Data Events: Register UI: Initialize UI: Front Panel State >> Open
        # "Initialization Macro\n(This is called once, when the VI starts)"
        n92 = call <vilib>:"Add State(s) to Queue__JKI_lib_State_Machine.vi"("State(s) in Front (\"\")"=w310, "State(s) in (\"\")"=w314) -> ("States Out"=w313:string)  [unwired: 13 in]
      }
      frame "Macro: Exit" {
        # "Exit Macro\n(This is called once, when the VI exits)"
        n93 = Unbundle By Name(w322) -> ("Core.Close Panel on Exit?"=w321:bool)
        n94 = Select(t="UI: Front Panel State >> Close", s=w321, f="") -> (s? t:f=w318:string)
        n95 = call <vilib>:"Add State(s) to Queue__JKI_lib_State_Machine.vi"("State(s) in (\"\")"=w318, "State(s) at Back (\"\")"="Data: Cleanup\nEvents: Unregister\nExit") -> ("States Out"=w316:string)  [unwired: 13 in]
        n96 = call <vilib>:"Add State(s) to Queue__JKI_lib_State_Machine.vi"("State(s) in Front (\"\")"=w316, "State(s) in (\"\")"=w325) -> ("States Out"=w324:string)  [unwired: 13 in]
      }
      frame "---------- API ----------" {
        # "Do not put any code in this frame.\n(It is a separator no-op. This category is recommanded to use for external API)"
      }
      frame "API: API1" {
        # "If you need to tell who triggered this state , use this string. If it's this case itself, this string is \"\"."
        # "Deal with the parameter if any"
        # "Connect this to return the response of your API"
        # "Copy/Rename this case for your own API"
      }
      frame "API: API2" {
        # "unpack HexStr  to Variant\nif complex parameter is needed."
        # "Copy/Rename this case for your own API"
        n97 = call "JKISM++ Convert HexStr to Data.vi"("HEX String"=w336) -> ()  [unwired: 8 in, 1 out]
        n98 = disable-structure shown="Disabled" {
          disable-tunnel: [w341 "API2 Response"] -> w335
          frame Disabled {
            # "pack variant to hexstr \nif complex response is needed."
            # "complex Response"
            n99 = call "JKISM++ Convert Data to HexStr.vi"() -> ("HEX String (0-9,A-F)"=w341:string)  [unwired: 9 in]
          }
          frame Enabled {
          }
        }
      }
      frame "---------- DoSth ----------" {
        # "Template Separator\n(You can make a copy of, or modify, this frame)"
        n100 = call <vilib>:"Add State(s) to Queue__JKI_lib_State_Machine.vi"("State(s) in (\"\")"=w347) -> ("States Out"=w346:string)  [unwired: 14 in]
      }
      frame "DoSth: DoA" {
        # "Your code here.\n(You can make a copy of, or modify, this frame)"
        n101 = call <vilib>:"Add State(s) to Queue__JKI_lib_State_Machine.vi"("State(s) in (\"\")"=w353) -> ("States Out"=w352:string)  [unwired: 14 in]
      }
      frame "DoSth: DoB" {
        # "Your code here.\n(You can make a copy of, or modify, this frame)"
        n102 = call <vilib>:"Add State(s) to Queue__JKI_lib_State_Machine.vi"("State(s) in (\"\")"=w359) -> ("States Out"=w358:string)  [unwired: 14 in]
      }
    }
  }
  n103 = call "Dispatch Worker.vi"("Name(\"\" to use uuid)"=w1) -> ()  [unwired: 11 in]
  n104 = call "Dispatch Worker.vi"("Name(\"\" to use uuid)"=w1) -> ()  [unwired: 11 in]
  n105 = call "Dispatch Worker.vi"("Name(\"\" to use uuid)"=w1) -> ()  [unwired: 11 in]
  n106 = call "Dispatch Worker.vi"("Name(\"\" to use uuid)"=w1) -> ()  [unwired: 11 in]
